vi "Send request (SubVI).vi"(4 "lockout_key":string, 5 "input json string":string, 7 "msgop":i32, 8 "error in (no error)":errorcluster, 10 "routing key":string, 11 "Exchange in":refnum<class "Exchange.lvclass">) -> (0 "error out":errorcluster, 3 "Exchange out":refnum<class "Exchange.lvclass">)   [LabVIEW 2016]
uses:
  <vilib>/Distrio/LabbitMQ/Exchange/Exchange.lvclass
  C:/Program Files/National Instruments/LabVIEW 2016/vi.lib/Distrio/LabbitMQ/RabbitMQ.Client.dll
panel:
  in  "ReplyTo":string="broadcast"
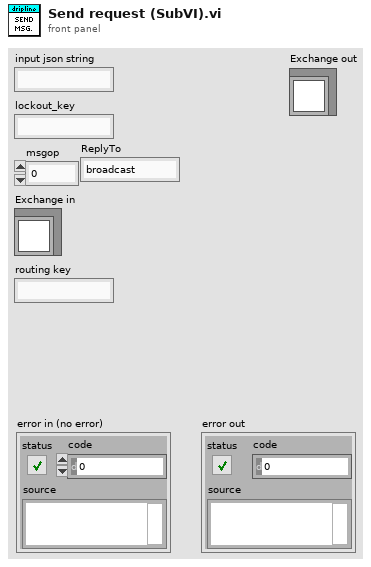
[diagram p1: front panel]
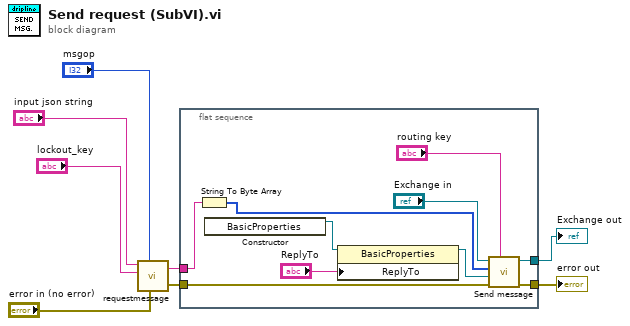
[diagram p0: block diagram]
diagram:
  n1 = call "requestmessage.vi"("error in (no error)"="error in (no error)", "msgop"="msgop", "lockout_key"="lockout_key", "input json string"="input json string") -> ("error out"=w8:errorcluster, "body"=w3:string)  [unwired: 2 in]
  n2 = flat-sequence {
    tunnel: w8 -> [w18]
    tunnel: [w17] -> w4
    tunnel: w3 -> [w15]
    tunnel: [w12] -> w2
    frame #0 {
      n3 = String To Byte Array(string=w15) -> (unsigned byte array=w16:u8[])
      n4 = constructor class="BasicProperties"() -> (reference out=w11:refnum<k24>)  [unwired: 3 in, 2 out]
      n5 = property class="BasicProperties"(reference=w11, "ReplyTo"="ReplyTo") -> (reference out=w9:refnum<k24>)  [unwired: 1 in, 1 out]
      n6 = call <vilib>:"Send message.vi"("routing key"="routing key", "error in (no error)"=w18, "MessageProperties"=w9, "body"=w16, "Exchange in"="Exchange in") -> ("error out"=w17:errorcluster, "Exchange out"=w12:refnum<class "Exchange.lvclass">)  [unwired: 5 in]
    }
  }
  "error out" <- w4
  "Exchange out" <- w2
